vi "Save_Destination_Type.vi"(8 "error in (no error)":errorcluster, 9 "index":string, 10 "buildObject":T1, 11 "IB_Destination in":refnum<class "IB_Destination.lvclass">) -> (0 "error out":errorcluster, 1 "index out":string, 2 "buildObject out":T1, 3 "IB_Destination out":refnum<class "IB_Destination.lvclass">)   [LabVIEW 2020, in "IB_Destination.lvclass"]
uses:
  <vilib>/AppBuilder/IB_Classes/Destination/IB_Destination.lvclass
  <vilib>/AppBuilder/IB_Classes/Destination/IB_Destination.lvclass/IB_Destination.ctl
  <resource>/Framework/Providers/API/ItemRef.ctl
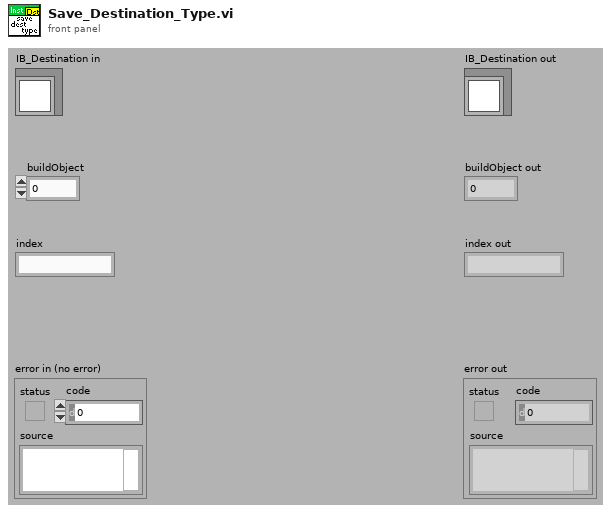
[diagram p1: front panel]
types:
  T1 = typedef "ItemRef.ctl" = u64
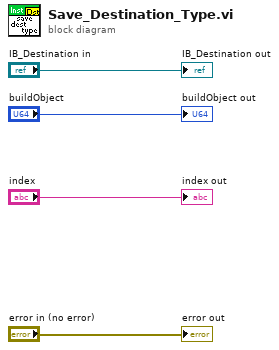
[diagram p0: block diagram]
diagram:
  "error out" <- "error in (no error)"
  "IB_Destination out" <- "IB_Destination in"
  "index out" <- "index"
  "buildObject out" <- "buildObject"
